vi "CarBody_CmdStr.vi"(1 "车身控制命令输入":T1 {"左前门锁状态" items=["未锁", "已锁", "预留", "错误"]; "左后门锁状态" items=["未锁", "已锁", "预留", "错误"]; "左后侧车窗位置状态" items=["中间位置", "完全打开", "完全关闭", "无效"]; "左后侧车窗运行状态" items=["停止", "手动升窗", "手动降窗", "自动升窗", "自动降窗", "预留"]; "左后侧车窗开度值" min=0 max=100 step=1 scale=0.0..100.0; "驾驶侧车窗位置状态" items=["中间位置", "完全打开", "完全关闭", "无效"]; "驾驶侧车窗运行状态" items=["停止", "手动升窗", "手动降窗", "自动升窗", "自动降窗", "预留"]; "驾驶侧车窗开度值" min=0 max=100 step=1 scale=0.0..100.0}) -> (0 "CmdStr":string)   [LabVIEW 2013]
uses:
  BCM_LDoor_285.ctl
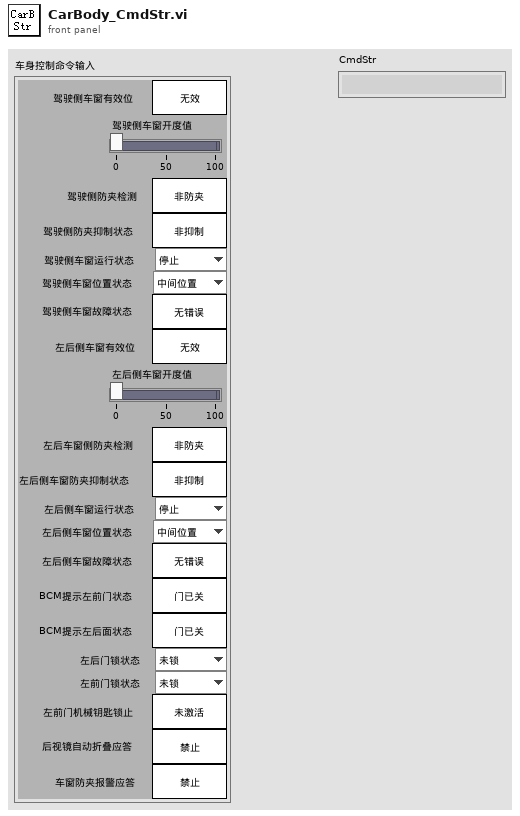
[diagram p1: front panel]
types:
  T1 = typedef "BCM_LDoor_285.ctl" = cluster{"驾驶侧车窗有效位":bool, "驾驶侧车窗开度值":i32, "驾驶侧防夹检测":bool, "驾驶侧防夹抑制状态":bool, "驾驶侧车窗运行状态":u16, "驾驶侧车窗位置状态":u16, "驾驶侧车窗故障状态":bool, "左后侧车窗有效位":bool, "左后侧车窗开度值":i32, "左后车窗侧防夹检测":bool, "左后侧车窗防夹抑制状态":bool, "左后侧车窗运行状态":u16, "左后侧车窗位置状态":u16, "左后侧车窗故障状态":bool, "BCM提示左前门状态":bool, "BCM提示左后面状态":bool, "左后门锁状态":u16, "左前门锁状态":u16, "左前门机械钥匙锁止":bool, "后视镜自动折叠应答":bool, "车窗防夹报警应答":bool}
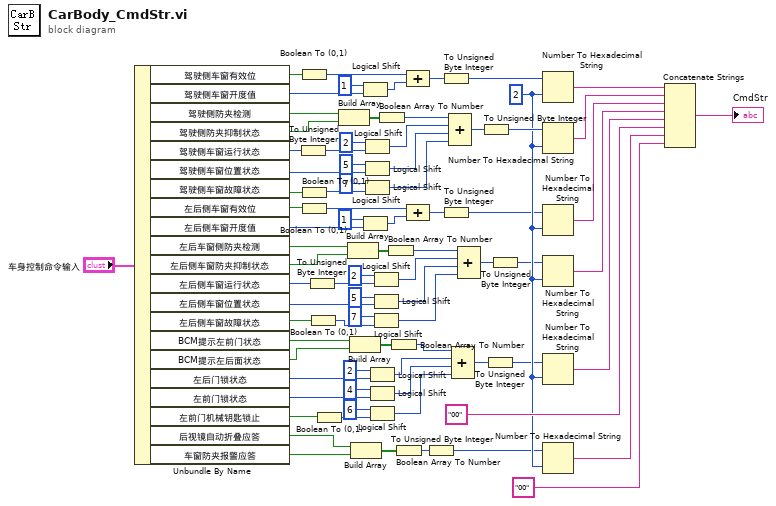
[diagram p0: block diagram]
diagram:
  w13 = 2
  n1 = Unbundle By Name("车身控制命令输入") -> ("驾驶侧车窗有效位"=w79:bool, "驾驶侧车窗开度值"=w78:i32, "驾驶侧防夹检测"=w73:bool, "驾驶侧防夹抑制状态"=w72:bool, "驾驶侧车窗运行状态"=w69:u16, "驾驶侧车窗位置状态"=w64:u16, "驾驶侧车窗故障状态"=w62:bool, "左后侧车窗有效位"=w53:bool, "左后侧车窗开度值"=w52:i32, "左后车窗侧防夹检测"=w42:bool, "左后侧车窗防夹抑制状态"=w41:bool, "左后侧车窗运行状态"=w40:u16, "左后侧车窗位置状态"=w39:u16, "左后侧车窗故障状态"=w38:bool, "BCM提示左前门状态"=w34:bool, "BCM提示左后面状态"=w33:bool, "左后门锁状态"=w31:u16, "左前门锁状态"=w27:u16, "左前门机械钥匙锁止"=w23:bool, "后视镜自动折叠应答"=w20:bool, "车窗防夹报警应答"=w19:bool)
  n2 = To Unsigned Byte Integer(number=w69) -> (unsigned 8bit integer=w65:u8)
  n3 = Boolean To (0,1)(Boolean=w79) -> (0, 1=w77:i16)
  n4 = Boolean To (0,1)(Boolean=w62) -> (0, 1=w61:i16)
  n5 = Boolean To (0,1)(Boolean=w53) -> (0, 1=w54:i16)
  n6 = To Unsigned Byte Integer(number=w40) -> (unsigned 8bit integer=w48:u8)
  n7 = Boolean To (0,1)(Boolean=w38) -> (0, 1=w37:i16)
  n8 = Boolean To (0,1)(Boolean=w23) -> (0, 1=w24:i16)
  n9 = Build Array(w73, w72) -> (w71:bool[])
  n10 = Build Array(w42, w41) -> (w43:bool[])
  n11 = Build Array(w34, w33) -> (w35:bool[])
  n12 = Build Array(w20, w19) -> (w18:bool[])
  n13 = Logical Shift(y=1, x=w78) -> (x << y=w76:i32)
  n14 = Logical Shift(y=1, x=w52) -> (x << y=w55:i32)
  n15 = Logical Shift(y=2, x=w65) -> (x << y=w66:u8)
  n16 = Logical Shift(y=5, x=w64) -> (x << y=w60:u16)
  n17 = Logical Shift(y=7, x=w61) -> (x << y=w59:i16)
  n18 = Logical Shift(y=2, x=w31) -> (x << y=w29:u16)
  n19 = Logical Shift(y=4, x=w27) -> (x << y=w25:u16)
  n20 = Logical Shift(y=6, x=w24) -> (x << y=w22:i16)
  n21 = Logical Shift(y=2, x=w48) -> (x << y=w47:u8)
  n22 = Logical Shift(y=5, x=w39) -> (x << y=w50:u16)
  n23 = Logical Shift(y=7, x=w37) -> (x << y=w36:i16)
  n24 = Boolean Array To Number(Boolean array=w71) -> (number=w68:u32)
  n25 = Boolean Array To Number(Boolean array=w43) -> (number=w45:u32)
  n26 = Boolean Array To Number(Boolean array=w35) -> (number=w30:u32)
  n27 = Boolean Array To Number(Boolean array=w18) -> (number=w17:u32)
  n28 = Compound Arithmetic op=ADD(w77, w76) -> (w75:i32)
  n29 = Compound Arithmetic op=ADD(w54, w55) -> (w56:i32)
  n30 = To Unsigned Byte Integer(number=w17) -> (unsigned 8bit integer=w3:u8)
  n31 = To Unsigned Byte Integer(number=w75) -> (unsigned 8bit integer=w15:u8)
  n32 = To Unsigned Byte Integer(number=w56) -> (unsigned 8bit integer=w6:u8)
  n33 = Compound Arithmetic op=ADD(w68, w66, w60, w59) -> (w58:u32)
  n34 = Compound Arithmetic op=ADD(w30, w29, w25, w22) -> (w21:u32)
  n35 = Compound Arithmetic op=ADD(w45, w47, w50, w36) -> (w51:u32)
  n36 = To Unsigned Byte Integer(number=w58) -> (unsigned 8bit integer=w14:u8)
  n37 = To Unsigned Byte Integer(number=w21) -> (unsigned 8bit integer=w4:u8)
  n38 = To Unsigned Byte Integer(number=w51) -> (unsigned 8bit integer=w5:u8)
  n39 = Number To Hexadecimal String(1:w13, 2:w15) -> (0:w12:string)
  n40 = Number To Hexadecimal String(1:w13, 2:w14) -> (0:w11:string)
  n41 = Number To Hexadecimal String(1:w13, 2:w6) -> (0:w10:string)
  n42 = Number To Hexadecimal String(1:w13, 2:w5) -> (0:w9:string)
  n43 = Number To Hexadecimal String(1:w13, 2:w4) -> (0:w8:string)
  n44 = Number To Hexadecimal String(1:w13, 2:w3) -> (0:w7:string)
  n45 = Concatenate Strings(w12, w11, w10, w9, w8, "00", w7, "00") -> (→"CmdStr":string)
